vi "picoscopeReadDataFromBuffer.vi"(5 "Data Pointers":T2, 6 "Sample Rate":sgl, 7 "Segment Range":T1 {"toSegmentIndex" format="%.4p"; "fromSegmentIndex" format="%.4p"}, 8 "error in (no error)":errorcluster, 9 "stop":bool, 10 "handle in":i16, 11 "PicoscopeV2 in":refnum<class "PicoscopeV2.lvclass">) -> (0 "error out":errorcluster, 1 "Trigger Offsets":cluster{u64, sgl}[](array[cluster]), 2 "MultiBuffers (Max or non-aggregated)":T3(array[cluster]), 3 "PicoscopeV2 out":refnum<class "PicoscopeV2.lvclass">)   [LabVIEW 2020, in "PicoscopeV2.lvclass"]
uses:
  PicoscopeV2.lvclass
  picosdk-ni-labview-examples-master/shared/PicoBuffers.ctl
  picosdk-ni-labview-examples-master/shared/Segment Range.ctl
  PicoscopeV2.lvclass/PicoscopeV2.ctl
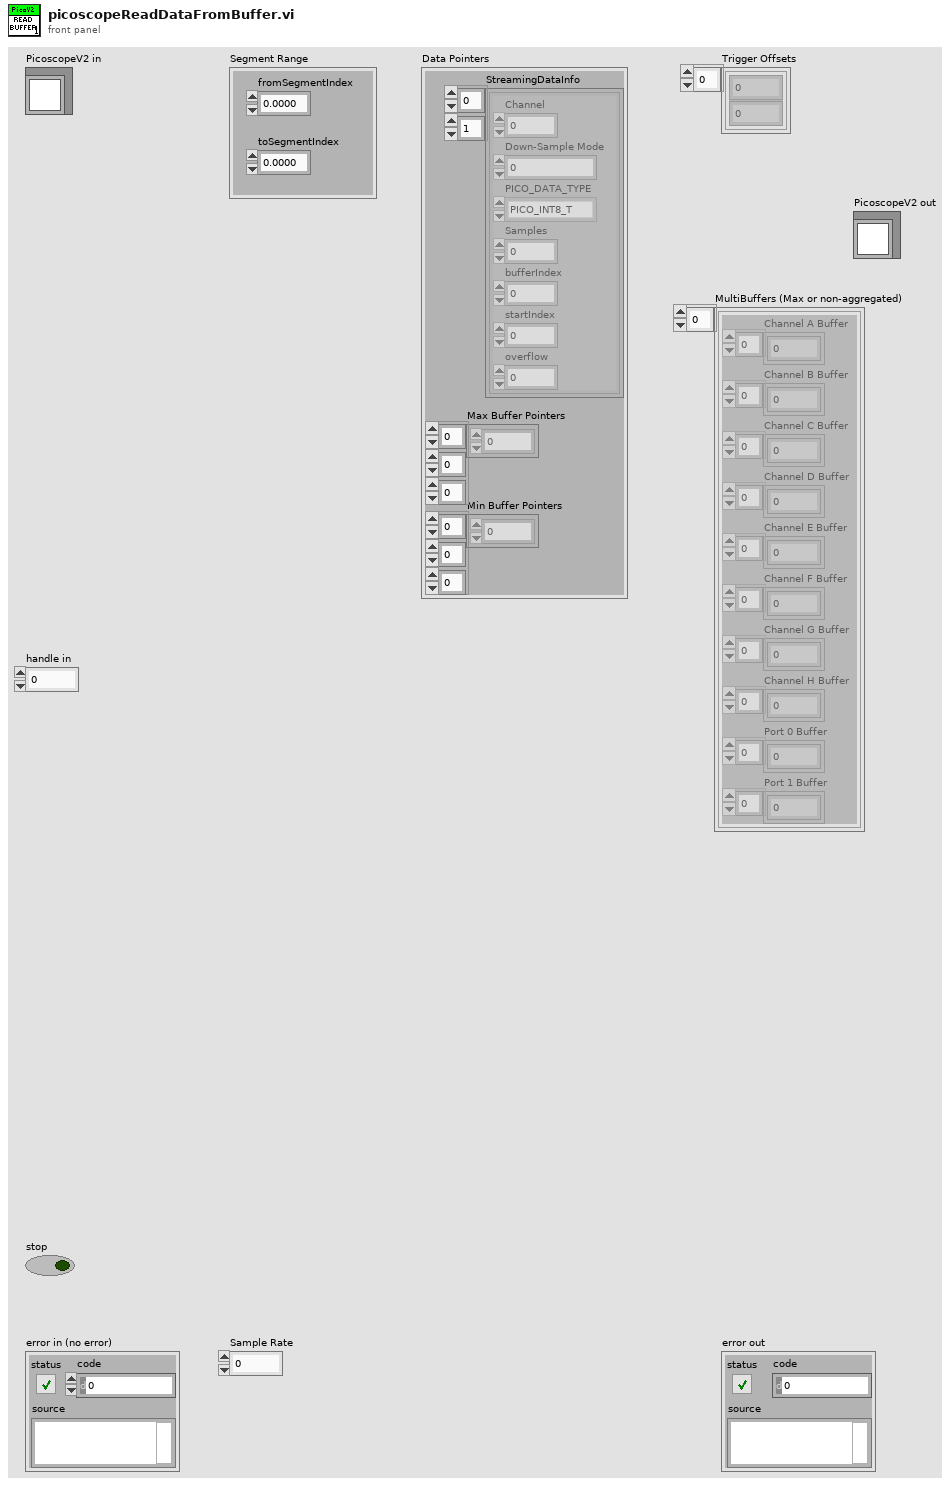
[diagram p1: front panel]
types:
  T1 = typedef "Segment Range.ctl" = cluster{"fromSegmentIndex":u64, "toSegmentIndex":u64}
  T2 = typedef "PicoBuffers.ctl" = cluster{"Max Buffer Pointers":u64[][][], "Min Buffer Pointers":u64[][][], "StreamingDataInfo":cluster{"Channel":u32, "Down-Sample Mode":u32, "PICO_DATA_TYPE":enum32{"PICO_INT8_T", "PICO_INT16_T", "PICO_INT32_T", "PICO_UINT32_T", "PICO_INT64_T", ""}, "Samples":i32, "bufferIndex":u64, "startIndex":i32, "overflow":i16}[][]}
  T3 = cluster{"Channel A Buffer":i16[], "Channel B Buffer":i16[], "Channel C Buffer":i16[], "Channel D Buffer":i16[], "Channel E Buffer":i16[], "Channel F Buffer":i16[], "Channel G Buffer":i16[], "Channel H Buffer":i16[], "Port 0 Buffer":i16[], "Port 1 Buffer":i16[]}[]
  T4 = typedef "Buffer and Transfer Settings.ctl" = cluster{"startIndex":u64, "Samples":u64, "Down Sample Ratio":u64, "Down-Sample Mode":u32}
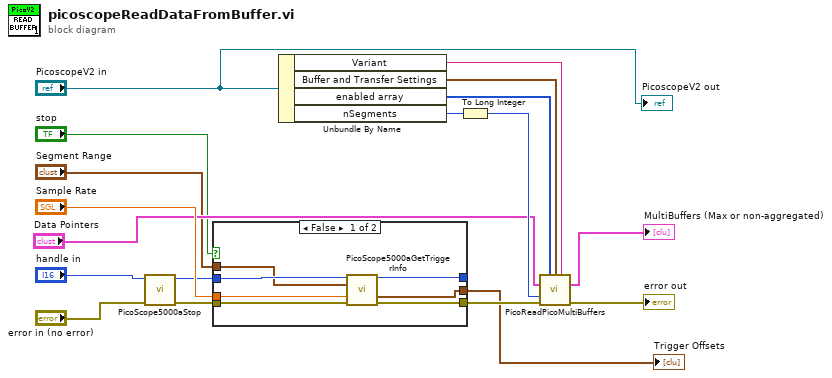
[diagram p0: block diagram]
diagram:
  n1 = call "PicoScope5000aStop.vi"("error in (no error)"="error in (no error)", "handle in"="handle in") -> ("error out"=w2:errorcluster, "handle out"=w3:i16)  [unwired: 8 in]
  n2 = case shown="False" "stop" {
    tunnel: [w25 w26] -> w10
    tunnel: [w24 w27] -> _
    tunnel: [w23 _] -> w8
    tunnel: w2 -> [w22 w26]
    tunnel: w3 -> [w21 w27]
    tunnel: "Segment Range" -> [w20 _]
    tunnel: "Sample Rate" -> [w19 _]
    frame False {
      n3 = call "PicoScope5000aGetTriggerInfo.vi"("handle in"=w21, "Rapid Block Acquisition Settings"=w20, "Sample Rate"=w19, "error in"=w22) -> ("handle out"=w24:i16, "Trigger Offsets"=w23:cluster{u64, sgl}[], "error out"=w25:errorcluster)  [unwired: 8 in, 1 out]
    }
    frame True {
    }
  }
  "Trigger Offsets" <- w8
  n4 = Unbundle By Name("PicoscopeV2 in") -> ("Variant"=w11:string, "Buffer and Transfer Settings"=w15:T4, "enabled array"=w12:i16[], "nSegments"=w13:i32)
  n5 = To Long Integer(number=w13) -> (32bit integer=w14:i32)
  n6 = call "PicoReadPicoMultiBuffers.vi"("enabled array"=w12, "Buffer and Transfer Settings"=w15, "Variant"=w11, "Data Pointers"="Data Pointers", "No of Buffers"=w14, "error in (no error)"=w10) -> ("MultiBuffers (Max or non-aggregated)"=→"MultiBuffers (Max or non-aggregated)":T3, "error out"=→"error out":errorcluster)  [unwired: 7 in, 1 out]
  "PicoscopeV2 out" <- "PicoscopeV2 in"
